vi "Register Application.vi"(10 "Application to Register":string) -> ()   [LabVIEW 2015, in "Reaper.lvclass"]
uses:
  Reaper.lvclass
  Reaper.lvclass/Reaper.ctl
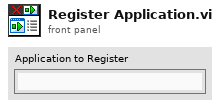
[diagram p1: front panel]
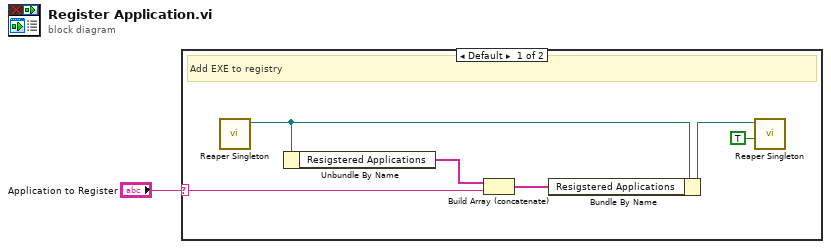
[diagram p0: block diagram]
diagram:
  n1 = case shown="Default" "Application to Register" {
    selector: "Application to Register" -> [w7 _]
    frame Default {
      # "Add EXE to registry"
      n2 = call "Reaper Singleton.vi"() -> ("Reaper Out"=w4:refnum<class "Reaper.lvclass">)  [unwired: 11 in]
      n3 = Unbundle By Name(w4) -> ("Resigstered Applications"=w6:string[])
      n4 = Build Array (concatenate)(w6, w7) -> (w5:string[])
      n5 = Bundle By Name(cluster=w4, "Resigstered Applications"=w5) -> (w2:refnum<class "Reaper.lvclass">)
      n6 = call "Reaper Singleton.vi"("Write? (F)"=TRUE, "Reaper In"=w2) -> ()  [unwired: 9 in, 1 out]
    }
    frame "" {
      # "No new EXE input -- Do nothing"
    }
  }
